vi "Music Visualizer Example.vi"() -> ()   [LabVIEW 2020]
doc: "A simple music visualizer.\n\nDemonstrates the G-Audio mixer and the mixed audio queue feature."
uses:
  Mixer/Mixer/Mixer.lvclass/Mixer.ctl
  <vilib>/Analysis/1siggen.llb/Ramp Pattern by Samples.vi
  <vilib>/Analysis/5stat.llb/RMS (DBL).vi
  Mixer/Mixer/Polymorphic VIs/Channel Load (Path).vi
  <vilib>/Analysis/NI_AALPro.lvlib
  <vilib>/ptbypt/NI_PtbyPt.lvlib
  <vilib>/Analysis/NI_AALBase.lvlib
  Mixer/Mixer/Mixer.lvclass
panel:
  in  "File Path":path
  in  "Size":dbl(slide)=1.0 scale=0.5..1.5
  in  "Color Box":u32(colorbox)=5883391
  in  "Stop":bool
  out "XY Graph":cluster{dbl[], dbl[]}[](graph)
  # "Instructions:\n1. Run the VI.\n2. Select an audio file to play using the path control.\n3. Use the controls to change the visualizer color and size.\n4. Press the Stop button to stop playback."
  # "+"
  # "-"
  # "G"
  # "-Audio"
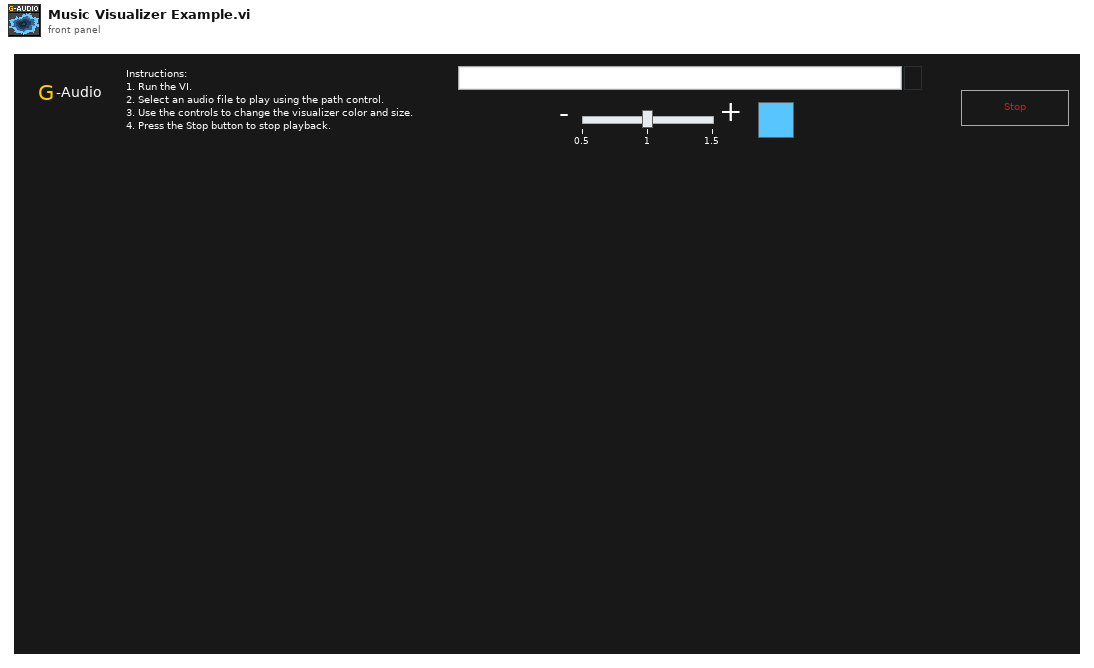
[diagram p1: front panel]
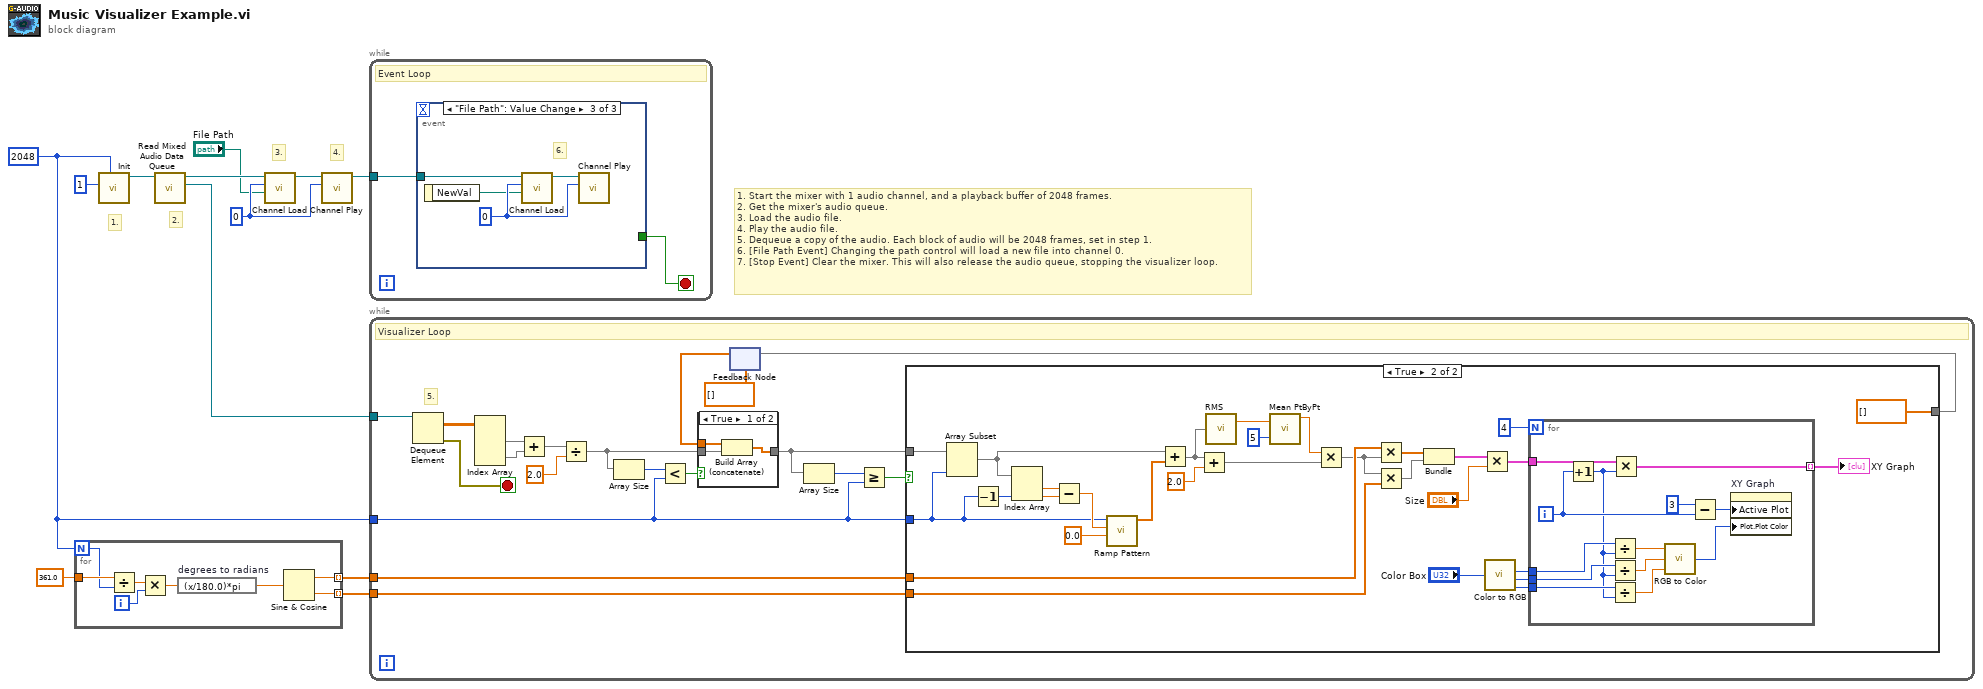
[diagram p0: block diagram]
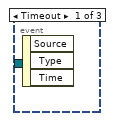
[diagram p4: hidden frame]
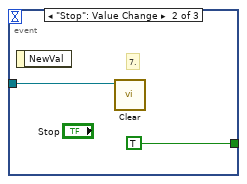
[diagram p5: hidden frame]
diagram:
  w9 = 0 ("Channel Index")
  w1 = 2048 ("Buffer Size (samples)")
  # "4."
  # "3."
  # "2."
  # "1."
  # "1. Start the mixer with 1 audio channel, and a playback buffer of 2048 frames.\n2. Get the mixer's audio queue.\n3. Load the audio file.\n4. Play the audio file.\n5. Dequeue a copy of the audio. Each block of audio will be 2048 frames, set in step 1.\n6. [File Path Event] Changing the path control will load a new file into channel 0.\n7. [Stop Event] Clear the mixer. This will also release the audio queue, stopping the visualizer loop."
  n1 = for {
    N: w1 -> [w19]
    tunnel: 361.0 -> [w20]
    tunnel: [w15] -> w2 mode=indexing
    tunnel: [w14] -> w3 mode=indexing
    i -> [w17]
    n2 = Divide(x=w20, y=w19) -> (x/y=w18:dbl)
    n3 = Multiply(x=w18, y=w17) -> (x*y=w16:dbl)
    n4 = expression code="(x/180.0)*pi" "degrees to radians"(w16) -> (w13:dbl)
    n5 = Sine & Cosine(0:w13) -> (1:w15:dbl, 2:w14:dbl)
  }
  n6 = call "Init.vi"("Playback Size (4096)"=w1, "Channel Count (16)"=1) -> ("Mixer out"=w5:refnum<class "Mixer.lvclass">)  [unwired: 8 in, 1 out]
  n7 = call "Read Mixed Audio Data Queue.vi"("Mixer in"=w5) -> ("Mixed Audio Data"=w4:refnum<queue>, "Mixer out"=w8:refnum<class "Mixer.lvclass">)  [unwired: 8 in, 1 out]
  n8 = call-poly "Channel Load.vi"("Path"="File Path", "Channel Index"=w9, "Mixer in"=w8) -> ("Mixer out"=w10:refnum<class "Mixer.lvclass">)  [unwired: 7 in, 1 out]
  n9 = call "Channel Play.vi"("Channel Index"=w9, "Mixer in"=w10) -> ("Mixer out"=w7:refnum<class "Mixer.lvclass">)  [unwired: 8 in, 1 out]
  n10 = while {
    tunnel: w7 -> [w22]
    stop <- w21 stop-if-true
    # "Event Loop"
    n11 = event shown="[2] \"File Path\": Value Change" {
      selector: _ -> [_ _ _]
      dyn-events: _ -> [_ _ _]
      timeout: _ -> [_ _ _]
      tunnel: w22 -> [_ w24 w26]
      tunnel: [_ TRUE _] -> w21
      event Timeout {
        n12 = event-data() -> ()  [unwired: 1 in, 3 out]
      }
      event "Stop": Value Change {
        # "7."
        n13 = event-data() -> ()  [unwired: 1 in, 1 out]
        n14 = call "Clear.vi"("Mixer in"=w24) -> ()  [unwired: 10 in, 1 out]
      }
      event "File Path": Value Change {
        w28 = 0 ("Channel Index")
        # "6."
        n15 = event-data() -> ("NewVal"=w25:path)  [unwired: 1 in]
        n16 = call-poly "Channel Load.vi"("Path"=w25, "Channel Index"=w28, "Mixer in"=w26) -> ("Mixer out"=w27:refnum<class "Mixer.lvclass">)  [unwired: 7 in, 1 out]
        n17 = call "Channel Play.vi"("Channel Index"=w28, "Mixer in"=w27) -> ()  [unwired: 8 in, 2 out]
      }
    }
  }
  n18 = while {
    tunnel: w2 -> [w47]
    tunnel: w3 -> [w46]
    tunnel: w4 -> [w45]
    tunnel: w1 -> [w38]
    stop <- w29 stop-if-true
    # "5."
    # "Visualizer Loop"
    n19 = Dequeue Element(queue=w45) -> (element=w35:dbl[][], error out=w29:errorcluster)  [unwired: 2 in, 2 out]
    n20 = Index Array(array=w35) -> (element #1=w34:dbl[], element #2=w33:dbl[])  [unwired: 4 in]
    n21 = Add(x=w34, y=w33) -> (x+y=w32:dbl[])
    n22 = Divide(x=w32, y=2.0) -> (x/y=w31:dbl[])
    n23 = Array Size(array=w31) -> (size(s)=w44:i32)
    n24 = Less?(x=w44, y=w38) -> (x < y?=w43:bool)
    n25 = feedback #1(dbl[] [] ("Audio Data")) -> (w42:dbl[])
    n26 = case shown="True" w43 {
      tunnel: w31 -> [w94 w95]
      tunnel: [w93 w95] -> w39
      tunnel: w42 -> [w92 _]
      frame True {
        n27 = Build Array (concatenate)(w92, w94) -> (w93:dbl[])
      }
      frame False {
      }
    }
    n28 = Array Size(array=w39) -> (size(s)=w41:i32)
    n29 = Greater Or Equal?(x=w41, y=w38) -> (x >= y?=w40:bool)
    n30 = case shown="True" w40 {
      tunnel: w47 -> [_ w78]
      tunnel: w46 -> [_ w77]
      tunnel: w39 -> [w48 w55]
      tunnel: w38 -> [_ w53]
      tunnel: [w48 dbl[] [] ("Audio Data")] -> w37
      frame False {
      }
      frame True {
        n31 = Array Subset(array=w55, length=w53) -> (w54:dbl[])  [unwired: 1 in]
        n32 = Decrement(x=w53) -> (x-1=w64:i32)
        n33 = Index Array(array=w54, index #2=w64) -> (element #1=w59:dbl, element #2=w60:dbl)  [unwired: 1 in]
        n34 = Subtract(x=w59, y=w60) -> (x-y=w61:dbl)
        n35 = call-poly <vilib>:"Ramp Pattern.vi"("start"=0.0, "end"=w61, "samples"=w53) -> ("Ramp Pattern"=w63:dbl[])  [unwired: 7 in, 1 out]
        n36 = Add(x=w54, y=w63) -> (x+y=w58:dbl[])
        n37 = Add(x=w58, y=2.0) -> (x+y=w76:dbl[])
        n38 = call-poly <vilib>:"RMS.vi"("X"=w58) -> ("rms value"=w67:dbl)  [unwired: 1 out]
        n39 = call <vilib>:"Mean PtByPt.vi"("x"=w67, "sample length"=5) -> ("mean"=w66:dbl)  [unwired: 2 in, 1 out]
        n40 = Multiply(x=w66, y=w76) -> (x*y=w68:dbl[])
        n41 = Multiply(x=w78, y=w68) -> (x*y=w74:dbl[])
        n42 = Multiply(x=w68, y=w77) -> (x*y=w73:dbl[])
        n43 = Bundle(w74, w73) -> (w57:cluster{dbl[], dbl[]})  [unwired: 1 in]
        n44 = Multiply(x=w57, y="Size") -> (x*y=w56:cluster{dbl[], dbl[]})
        n45 = call <vilib>:"Color to RGB.vi"("Color"="Color Box") -> ("R"=w71:u8, "G"=w70:u8, "B"=w69:u8)  [unwired: 1 out]
        n46 = for {
          N: 4 -> [_]
          tunnel: w56 -> [w91]
          tunnel: [w90] -> w51 mode=indexing
          tunnel: w71 -> [w88]
          tunnel: w70 -> [w87]
          tunnel: w69 -> [w86]
          i -> [w89]
          n47 = Increment(x=w89) -> (x+1=w85:i32)
          n48 = Divide(x=w88, y=w85) -> (x/y=w83:dbl)
          n49 = Divide(x=w87, y=w85) -> (x/y=w82:dbl)
          n50 = Divide(x=w86, y=w85) -> (x/y=w84:dbl)
          n51 = Multiply(x=w91, y=w85) -> (x*y=w90:cluster{dbl[], dbl[]})
          n52 = call <vilib>:"RGB to Color.vi"("B"=w84, "G"=w82, "R"=w83) -> ("Color"=w79:u32)
          n53 = Subtract(x=3, y=w89) -> (x-y=w80:i32)
          n54 = property on="XY Graph" class="XYGraph (strict)"("Active Plot"=w80, "Plot.Plot Color"=w79) -> ()  [unwired: 2 in, 2 out]
        }
        "XY Graph" <- w51
      }
    }
    n55 = feedback-in #1(w37) -> ()
  }
